vi "Sync scrollbars.vi"(7 "Min cursor moved":bool, 8 "error in (no error)":errorcluster, 11 "Scrollbar value":i32) -> (0 "error out":errorcluster)   [LabVIEW 2020]
uses:
  Globals/gl_Time series viewer globals.vi
panel:
  out "Extractor slider":cluster{"Min cursor":i32, "Max cursor":i32}
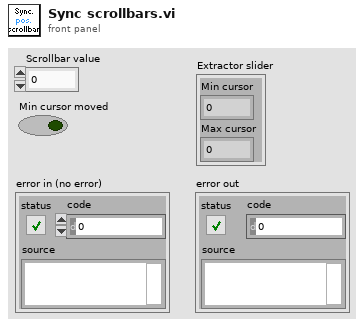
[diagram p1: front panel]
types:
  T1 = typedef "Time series viewer refs.ctl" = cluster{"This VI":refnum<vi>, "Image control":refnum<vi>, "AVI Mode ind":refnum<vi>, "Play":refnum<vi>, "Stop":refnum<vi>, "Back":refnum<vi>, "Scrollbar":refnum<vi>, "Video length info":refnum<vi>, "Expected speed values":refnum<vi>, "Intensity":refnum<vi>, "Path":refnum<vi>, "Selection sliders":refnum<vi>, "Speed Graph ref":refnum<vi>, "Frame rate set (fps)":refnum<vi>, "Number of rows to generate":refnum<vi>, "VL Image Array":refnum<vi>, "Image Scrollbar":refnum<vi>, "Channel to load":refnum<vi>, "Colour":refnum<vi>}
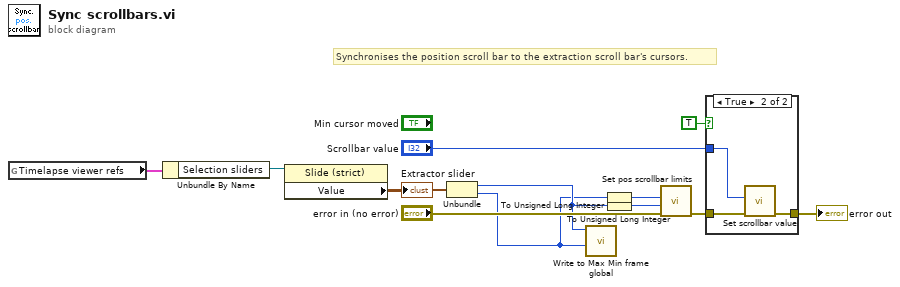
[diagram p0: block diagram]
diagram:
  # "Synchronises the position scroll bar to the extraction scroll bar's cursors."
  n1 = global read "gl_Time series viewer globals.vi" "Timelapse viewer refs"() -> (w4:T1)
  n2 = Unbundle By Name(w4) -> ("Selection sliders"=w3:refnum<vi>)
  n3 = property class="Slide (strict)"(reference=w3) -> ("Value"=w2:cluster{i32, i32})  [unwired: 1 in, 2 out]
  "Extractor slider" <- w2
  n4 = Unbundle(w2) -> (w8:i32, w1:i32)
  n5 = call "Write to Max Min frame global.vi"("Max cursor / End frame"=w1, "Min cursor / Start frame"=w8) -> ()  [unwired: 10 in]
  n6 = To Unsigned Long Integer(number=w1) -> (unsigned 32bit integer=w6:u32)
  n7 = To Unsigned Long Integer(number=w8) -> (unsigned 32bit integer=w5:u32)
  n8 = call "Set pos scrollbar limits.vi"("error in (no error)"="error in (no error)", "Min frame (unity-based)"=w5, "Max frame (unity-based)"=w6) -> ("error out"=w11:errorcluster)  [unwired: 8 in]
  n9 = case shown="True" TRUE {
    tunnel: "Scrollbar value" -> [_ w16]
    tunnel: w11 -> [w13 w15]
    tunnel: [w13 w14] -> w10
    frame False {
    }
    frame True {
      n10 = call "Set scrollbar value.vi"("error in (no error)"=w15, "Scrollbar value"=w16) -> ("error out"=w14:errorcluster)  [unwired: 9 in]
    }
  }
  "error out" <- w10
